vi "Set Digital Offset.vi"(0 "gen in":refnum<class "niUSRP Tx DSP v2 FPGA.lvclass">, 1 "channel":u8, 5 "digital offset":refnum<class "Digital Offset Interface (IQ 18-bit).lvclass">) -> (4 "gen out":refnum<class "niUSRP Tx DSP v2 FPGA.lvclass">)   [LabVIEW 2025, in "niUSRP Tx DSP v2 FPGA.lvclass"]
uses:
  niUSRP Tx DSP v2 FPGA.lvclass
  <instrlib>/_niInstr/DSP Control/Interface/v1/FPGA/Digital Offset/IQ 18-bit/Digital Offset Interface (IQ 18-bit).lvclass
  niUSRP Tx DSP v2 FPGA.lvclass/niUSRP Tx DSP v2 FPGA.ctl
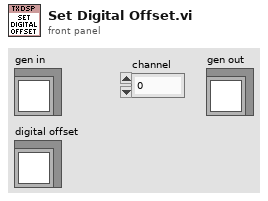
[diagram p1: front panel]
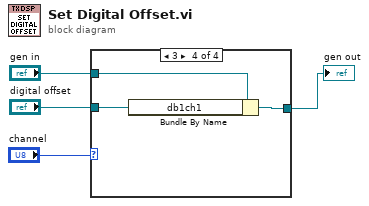
[diagram p0: block diagram]
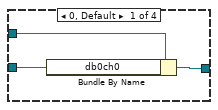
[diagram p2: hidden frame]
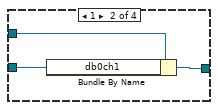
[diagram p3: hidden frame]
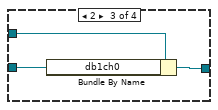
[diagram p4: hidden frame]
diagram:
  n1 = case shown="3" "channel" {
    tunnel: "gen in" -> [w7 w10 w13 w16]
    tunnel: [w6 w9 w12 w15] -> w3
    tunnel: "digital offset" -> [w5 w8 w11 w14]
    frame 0, Default {
      n2 = Bundle By Name(cluster=w7, "db0ch0"=w5) -> (w6:refnum<class "niUSRP Tx DSP v2 FPGA.lvclass">)
    }
    frame 1 {
      n3 = Bundle By Name(cluster=w10, "db0ch1"=w8) -> (w9:refnum<class "niUSRP Tx DSP v2 FPGA.lvclass">)
    }
    frame 2 {
      n4 = Bundle By Name(cluster=w13, "db1ch0"=w11) -> (w12:refnum<class "niUSRP Tx DSP v2 FPGA.lvclass">)
    }
    frame 3 {
      n5 = Bundle By Name(cluster=w16, "db1ch1"=w14) -> (w15:refnum<class "niUSRP Tx DSP v2 FPGA.lvclass">)
    }
  }
  "gen out" <- w3
